vi "cyclic buffer.vi"(9 "dimension size":i32, 10 "new element":cdb) -> (2 "delayed \nelement":cdb)   [LabVIEW 2017]
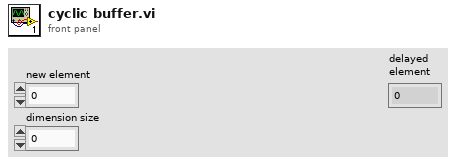
[diagram p1: front panel]
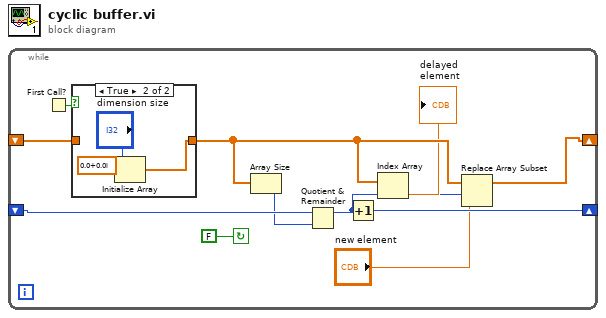
[diagram p0: block diagram]
diagram:
  n1 = while {
    shift-right: [w8] -> _
    shift-left: _ -> [w9]
    shift-right: [w4] -> _
    shift-left: _ -> [w7]
    stop <- FALSE continue-if-true
    n2 = First Call?() -> (First Call?: T/F=w10:bool)
    n3 = case shown="True" w10 {
      tunnel: [w12 w15] -> w6
      tunnel: w9 -> [w12 _]
      frame False {
      }
      frame True {
        n4 = Initialize Array(cdb 0.0+0.0i ("element"), "dimension size") -> (w15:cdb[])
      }
    }
    n5 = Array Size(array=w6) -> (size(s)=w5:i32)
    n6 = Quotient & Remainder(x=w7, y=w5) -> (x-y*floor(x/y)=w1:i32)  [unwired: 1 out]
    n7 = Increment(x=w1) -> (x+1=w4:i32)
    n8 = Index Array(array=w6, index=w1) -> (element=→"delayed \nelement":cdb)
    n9 = Replace Array Subset(array=w6, new element="new element", index=w1) -> (w8:cdb[])
  }
